vi "EndOfTrain.vi"() -> ()   [LabVIEW 2019]
panel:
  in  "OK Button":bool
  # "Zakoñczono Trening"
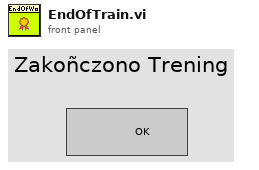
[diagram p1: front panel]
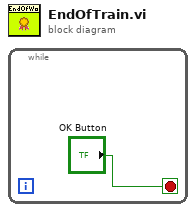
[diagram p0: block diagram]
diagram:
  n1 = while {
    stop <- "OK Button" stop-if-true
  }
